vi "Read Launch Button.vi"(11 "array":bool[](array[boolean])) -> ()   [LabVIEW 2020]
uses:
  Robot Global Data.vi
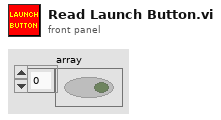
[diagram p1: front panel]
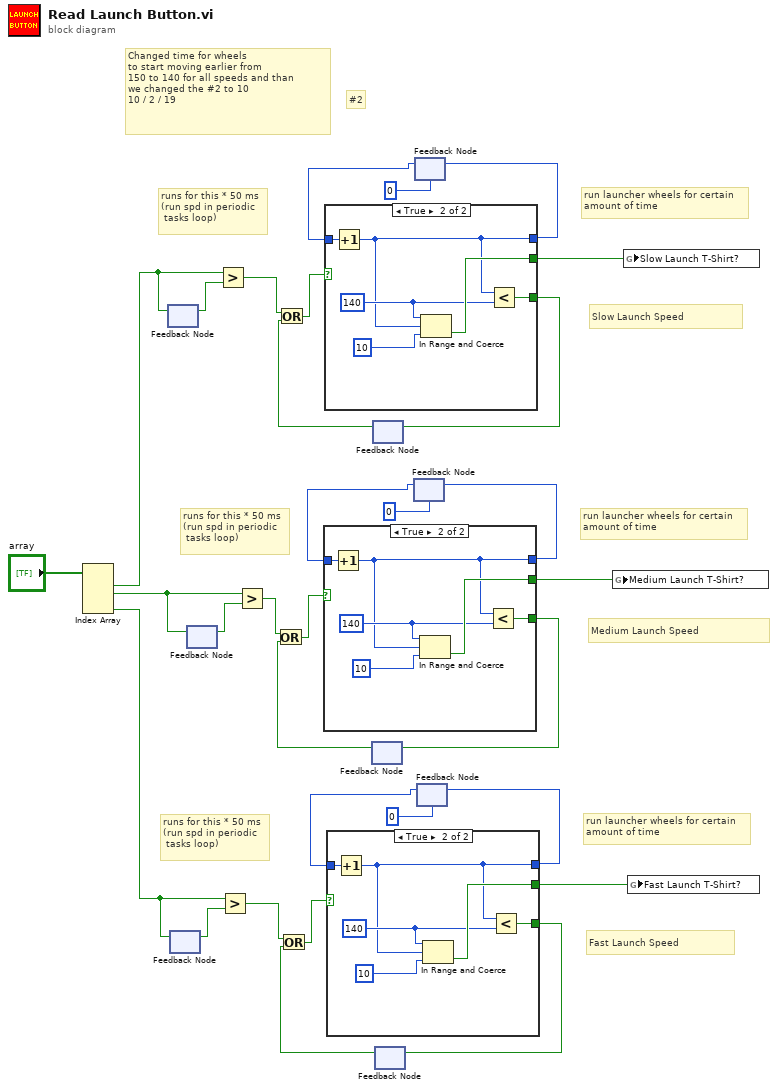
[diagram p0: block diagram]
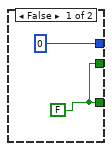
[diagram p2: hidden frame]
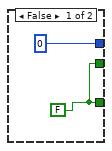
[diagram p3: hidden frame]
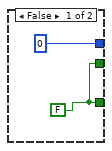
[diagram p4: hidden frame]
diagram:
  # "#2"
  # "Changed time for wheels\nto start moving earlier from\n150 to 140 for all speeds and than\nwe changed the #2 to 10\n10 / 2 / 19"
  # "Fast Launch Speed"
  # "Medium Launch Speed"
  # "Slow Launch Speed"
  # "runs for this * 50 ms\n(run spd in periodic\n tasks loop)"
  # "run launcher wheels for certain\namount of time"
  # "runs for this * 50 ms\n(run spd in periodic\n tasks loop)"
  # "run launcher wheels for certain\namount of time"
  # "runs for this * 50 ms\n(run spd in periodic\n tasks loop)"
  # "run launcher wheels for certain\namount of time"
  n1 = Index Array(array="array") -> (element #1=w31:bool, element #2=w2:bool, element #4=w1:bool)  [unwired: 4 in, 1 out]
  n2 = feedback #1() -> (w30:bool)  [unwired: 1 in]
  n3 = feedback-in #1(w31) -> ()
  n4 = feedback #2() -> (w11:bool)  [unwired: 1 in]
  n5 = feedback-in #2(w1) -> ()
  n6 = feedback #3() -> (w20:bool)  [unwired: 1 in]
  n7 = feedback-in #3(w2) -> ()
  n8 = Greater?(x=w31, y=w30) -> (0:w28:bool)
  n9 = Greater?(x=w1, y=w11) -> (0:w9:bool)
  n10 = Greater?(x=w2, y=w20) -> (0:w18:bool)
  n11 = feedback #4() -> (w17:bool)  [unwired: 1 in]
  n12 = Or(x=w18, y=w17) -> (x .or. y?=w19:bool)
  n13 = feedback #5() -> (w27:bool)  [unwired: 1 in]
  n14 = Or(x=w28, y=w27) -> (x .or. y?=w29:bool)
  n15 = feedback #6() -> (w8:bool)  [unwired: 1 in]
  n16 = Or(x=w9, y=w8) -> (x .or. y?=w10:bool)
  n17 = feedback #7(0) -> (w15:i32)
  n18 = case shown="True" w19 {
    tunnel: w15 -> [_ w39]
    tunnel: [0 w35] -> w14
    tunnel: [w32 w38] -> w13
    tunnel: [w32 w37] -> w12
    frame False {
      w32 = FALSE
    }
    frame True {
      w36 = 140 ("Time to Shoot")
      n19 = Increment(x=w39) -> (x+1=w35:i32)
      n20 = In Range and Coerce(upper limit=w36, x=w35, lower limit=10) -> (In Range?=w37:bool)  [unwired: 1 out]
      n21 = Less?(x=w35, y=w36) -> (x < y?=w38:bool)
    }
  }
  n22 = feedback-in #4(w13) -> ()
  n23 = feedback-in #7(w14) -> ()
  n24 = feedback #8(0) -> (w25:i32)
  n25 = case shown="True" w29 {
    tunnel: w25 -> [_ w47]
    tunnel: [0 w43] -> w24
    tunnel: [w40 w46] -> w23
    tunnel: [w40 w45] -> w21
    frame False {
      w40 = FALSE
    }
    frame True {
      w44 = 140 ("Time to Shoot")
      n26 = Increment(x=w47) -> (x+1=w43:i32)
      n27 = In Range and Coerce(upper limit=w44, x=w43, lower limit=10) -> (In Range?=w45:bool)  [unwired: 1 out]
      n28 = Less?(x=w43, y=w44) -> (x < y?=w46:bool)
    }
  }
  n29 = feedback-in #5(w23) -> ()
  n30 = feedback-in #8(w24) -> ()
  n31 = feedback #9(0) -> (w6:i32)
  n32 = case shown="True" w10 {
    tunnel: w6 -> [_ w55]
    tunnel: [0 w51] -> w5
    tunnel: [w48 w54] -> w4
    tunnel: [w48 w53] -> w3
    frame False {
      w48 = FALSE
    }
    frame True {
      w52 = 140 ("Time to Shoot")
      n33 = Increment(x=w55) -> (x+1=w51:i32)
      n34 = In Range and Coerce(upper limit=w52, x=w51, lower limit=10) -> (In Range?=w53:bool)  [unwired: 1 out]
      n35 = Less?(x=w51, y=w52) -> (x < y?=w54:bool)
    }
  }
  n36 = feedback-in #6(w4) -> ()
  n37 = feedback-in #9(w5) -> ()
  n38 = global write "Robot Global Data.vi" "Medium Launch T-Shirt?"(w12) -> ()
  n39 = global write "Robot Global Data.vi" "Slow Launch T-Shirt?"(w21) -> ()
  n40 = global write "Robot Global Data.vi" "Fast Launch T-Shirt?"(w3) -> ()
